vi "ProcessCalibrationData.vi"(7 "connection ID":refnum<k5>, 10 "Fiducial 2":dbl[][](array[numeric]), 11 "Fiducial 1":dbl[][](array[numeric])) -> ()   [LabVIEW 2018]
uses:
  <vilib>/Analysis/baseanly.llb/Mean (DBL).vi
  <vilib>/Utility/file.llb/Write Delimited Spreadsheet (DBL).vi
  <vilib>/Analysis/NI_AALBase.lvlib
panel:
  out "Average Length":dbl format="%_8g"
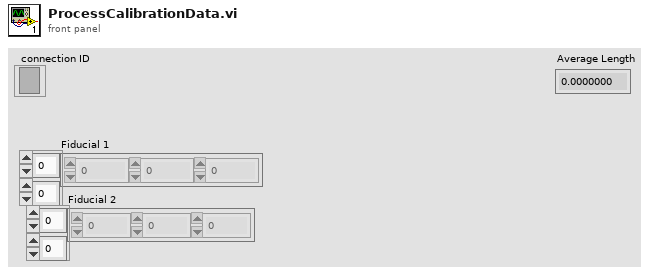
[diagram p1: front panel]
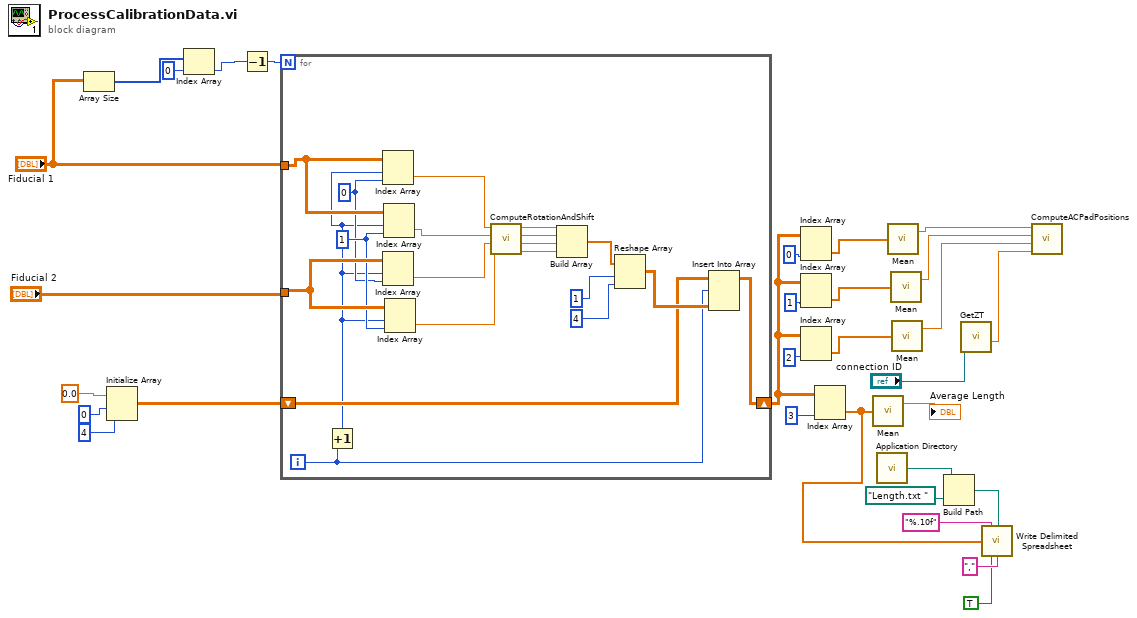
[diagram p0: block diagram]
diagram:
  n1 = Array Size(array="Fiducial 1") -> (size(s)=w26:i32[])
  n2 = Initialize Array(0.0 ("element"), 0 ("dimension size"), 4 ("dimension size")) -> (w24:dbl[][])
  n3 = Index Array(array=w26, index=0) -> (element=w2:i32)
  n4 = Decrement(x=w2) -> (x-1=w1:i32)
  n5 = for {
    N: w1 -> [_]
    tunnel: "Fiducial 1" -> [w51]
    tunnel: "Fiducial 2" -> [w50]
    shift-right: [w39] -> w14
    shift-left: w24 -> [w38]
    i -> [w40]
    w49 = 1 ("disabled index (col)")
    w48 = 0 ("disabled index (col)")
    n6 = Increment(x=w40) -> (x+1=w32:i32)
    n7 = Index Array(array=w51, index (row)=w32, index (col)=w48) -> (element=w47:dbl)
    n8 = Index Array(array=w50, index (row)=w32, index (col)=w48) -> (element=w45:dbl)
    n9 = Index Array(array=w51, index (row)=w32, index (col)=w49) -> (element=w46:dbl)
    n10 = Index Array(array=w50, index (row)=w32, index (col)=w49) -> (element=w44:dbl)
    n11 = call "ComputeRotationAndShift.vi"("Y2"=w44, "X2"=w45, "Y1"=w46, "X1"=w47) -> ("Length"=w33:dbl, "YShift"=w35:dbl, "XShift"=w36:dbl, "Theta (Rad)"=w37:dbl)  [unwired: 4 in]
    n12 = Build Array(w37, w36, w35, w33) -> (w42:dbl[])
    n13 = Reshape Array(w42, 1 ("dimension size"), 4 ("dimension size")) -> (w43:dbl[][])
    n14 = Insert Into Array(array=w38, index (row)=w40, new element=w43) -> (w39:dbl[][])  [unwired: 1 in]
  }
  n15 = Index Array(array=w14, index (col)=0 ("disabled index (col)")) -> (element=w23:dbl[])  [unwired: 1 in]
  n16 = Index Array(array=w14, index (col)=1 ("disabled index (col)")) -> (element=w22:dbl[])  [unwired: 1 in]
  n17 = Index Array(array=w14, index (col)=2 ("disabled index (col)")) -> (element=w21:dbl[])  [unwired: 1 in]
  n18 = Index Array(array=w14, index (col)=3 ("disabled index (col)")) -> (element=w4:dbl[])  [unwired: 1 in]
  n19 = call-poly <vilib>:"Mean.vi"("X"=w4) -> ("mean"=→"Average Length":dbl)  [unwired: 1 out]
  n20 = call <vilib>:"Application Directory.vi"() -> ("Application Directory"=w8:path)
  n21 = call-poly <vilib>:"Mean.vi"("X"=w23) -> ("mean"=w17:dbl)  [unwired: 1 out]
  n22 = call-poly <vilib>:"Mean.vi"("X"=w22) -> ("mean"=w16:dbl)  [unwired: 1 out]
  n23 = call-poly <vilib>:"Mean.vi"("X"=w21) -> ("mean"=w15:dbl)  [unwired: 1 out]
  n24 = Build Path(base path=w8, name or relative path=path "Length.txt " ("file path (dialog if empty)")) -> (appended path=w7:path)
  n25 = call "GetZT.vi"("connection ID"="connection ID") -> ("Theta (rad)"=w11:dbl)  [unwired: 7 in, 3 out]
  n26 = call-poly <vilib>:"Write Delimited Spreadsheet.vi"("file path (dialog if empty)"=w7, "format (%.3f)"="%.10f", "1D data"=w4, "transpose? (no:F)"=TRUE, "delimiter (\\t)"="," ("delimiter (\\t)")) -> ()  [unwired: 9 in, 2 out]
  n27 = call "ComputeACPadPositions.vi"("Theta Calibration"=w17, "X cp"=w16, "Y cp"=w15, "Stage Initial\nRotation"=w11) -> ()  [unwired: 7 in]
